vi "exercise7_readAI_samplesloop.vi"() -> ()   [LabVIEW 2018]
uses:
  <vilib>/DAQmx/read.llb/DAQmx Read (Analog Wfm 1Chan NSamp).vi
  <vilib>/DAQmx/create/channels.llb/DAQmx Create Channel (AI-Voltage-Basic).vi
  <vilib>/DAQmx/configure/timing.llb/DAQmx Timing (Sample Clock).vi
  <vilib>/DAQmx/miscellaneous.llb/DAQmx Fill In Error Info.vi
  <vilib>/express/express analysis/Spectral/Block/exnSpectralBlock spectral measurements RMS poly.vi
  <vilib>/express/express analysis/Spectral/Block/exnSpectralBlock spectral measurements RMS array WFM.vi
  <vilib>/express/express analysis/Spectral/XNode/ExpressSpectralMeasurementsBlockNode.xnode
panel:
  out "Waveform Chart (Pa)":waveform(dbl)(graph)
  out "FFT":cluster{"f0":dbl, "df":dbl, "magnitude":dbl[]}[](graph)
  in  "?":bool
  in  "maximum value":dbl=5.0
  in  "minimum value":dbl=-5.0
  in  "sample mode":i32(ring)=10123 items=["Finite Samples"=10178, "Continuous Samples"=10123, "Hardware Timed Single Point"=12522]
  in  "samples per channel":i32=40
  in  "rate":dbl=20.0
  out "error out":errorcluster
  out "Waveform Graph":waveform(dbl)(graph)
  out "Waveform Chart":waveform(dbl)(graph)
  in  "NI_channels":tag="Dev1/ai0"
  # "CANAL 0"
  # "CANAL 0"
  # "ACQUIRE SIGNAL (CONTINUOUS)"
  # "CHANNEL CONFIG"
  # "SAMPLING CONFIG"
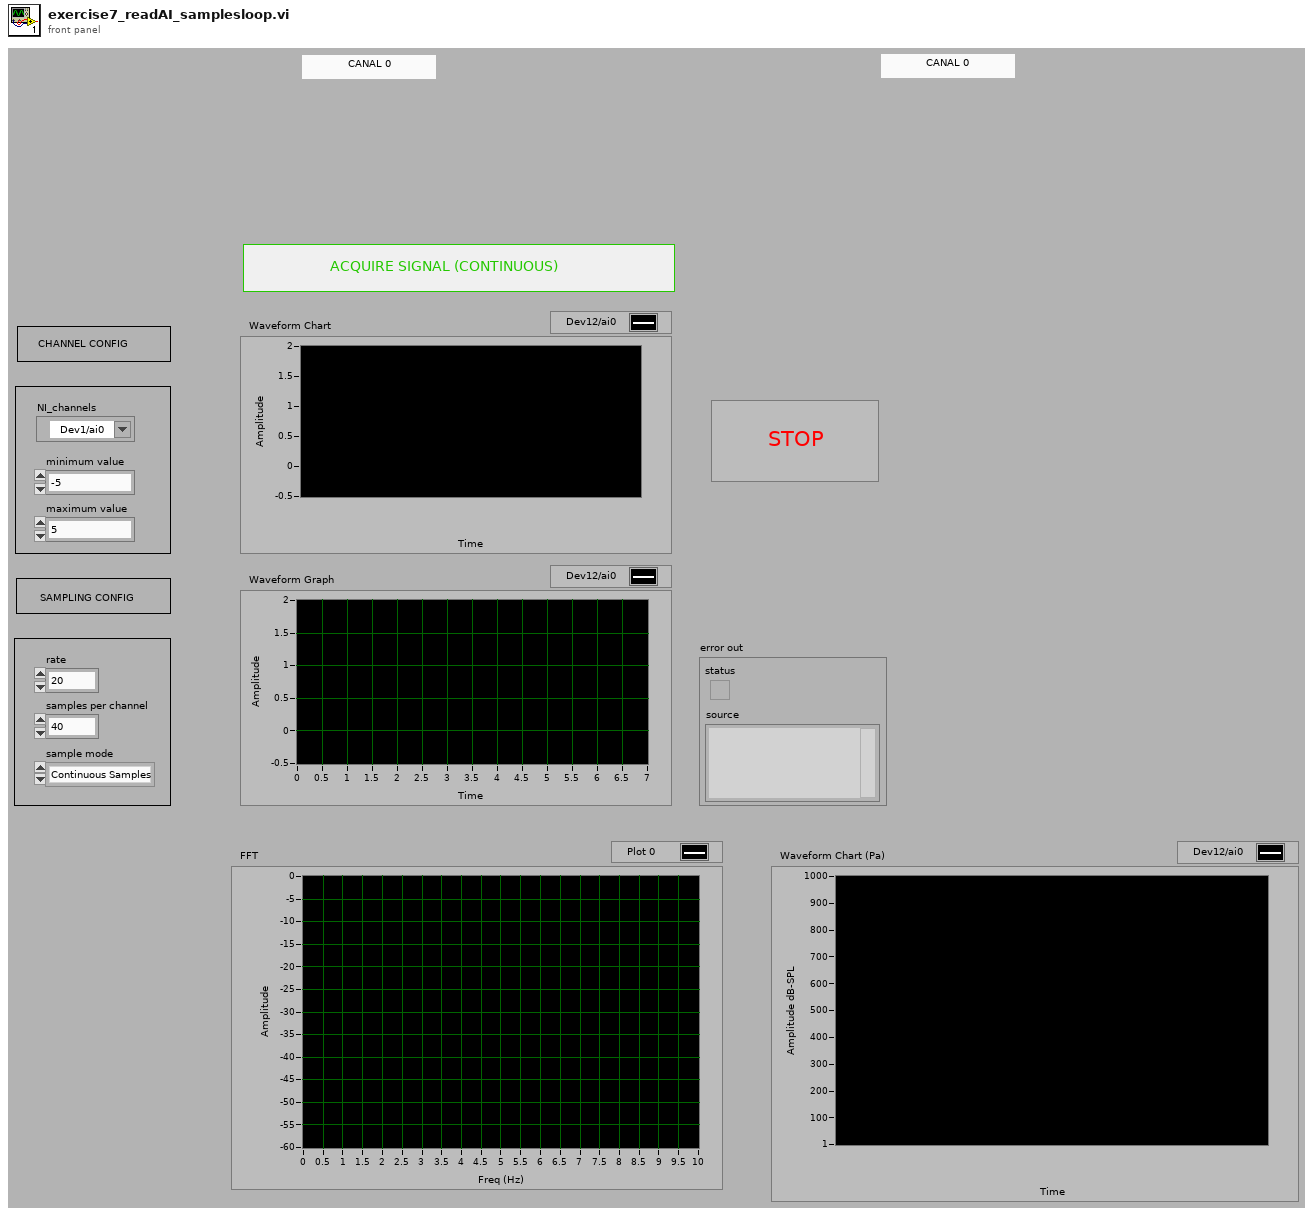
[diagram p1: front panel]
types:
  T1 = cluster{"averaging mode":u16, "weighting mode":u16, "number of averages":u32}
  T2 = cluster{"dB On (F)":bool, "unwrap phase (F)":bool, "convert to degree (F)":bool}
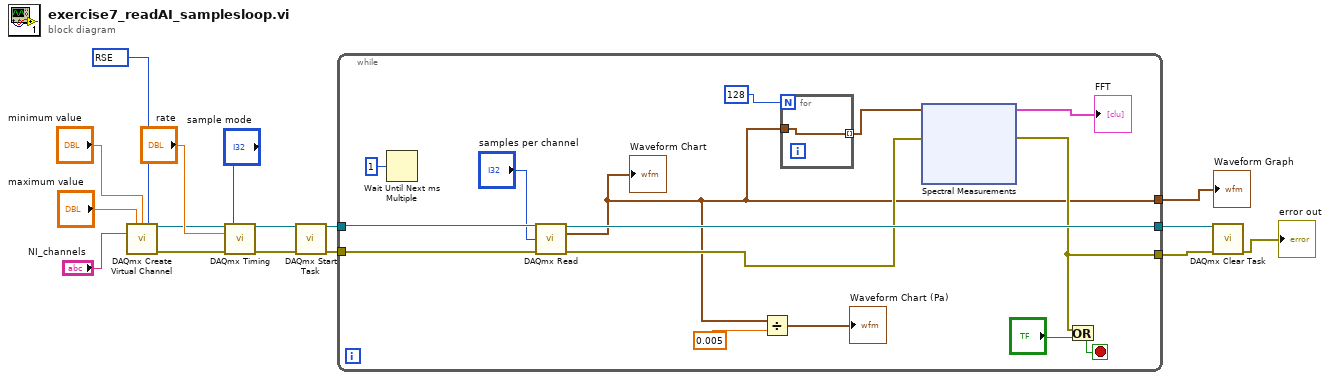
[diagram p0: block diagram]
diagram:
  w4 = 10083 items=["default"=-1, "RSE"=10083, "NRSE"=10078, "Differential"=10106, "Pseudodifferential"=12529] ("input terminal configuration")
  n1 = call-poly <vilib>:"DAQmx Create Virtual Channel.vi"("maximum value"="maximum value", "minimum value"="minimum value", "input terminal configuration"=w4, "physical channels"="NI_channels") -> ("task out"=w14:refnum<k21>, "error out"=w13:errorcluster)  [unwired: 10 in]
  n2 = call-poly <vilib>:"DAQmx Timing.vi"("task/channels in"=w14, "sample mode"="sample mode", "rate"="rate", "error in"=w13) -> ("task out"=w9:refnum<k21>, "error out"=w8:errorcluster)  [unwired: 10 in]
  n3 = call <vilib>:"DAQmx Start Task.vi"("task/channels in"=w9, "error in"=w8) -> ("task out"=w6:refnum<k21>, "error out"=w7:errorcluster)  [unwired: 12 in]
  n4 = while {
    tunnel: w7 -> [w31]
    tunnel: w6 -> [w30]
    tunnel: [w19] -> w3
    tunnel: [w29] -> w5
    tunnel: [w20] -> w2
    stop <- w26 stop-if-true
    n5 = Wait Until Next ms Multiple(millisecond multiple=u32 1) -> ()  [unwired: 1 out]
    n6 = call-poly <vilib>:"DAQmx Read.vi"("task/channels in"=w30, "number of samples per channel"="samples per channel", "error in"=w31) -> ("task out"=w29:refnum<k21>, "data"=w19:waveform(dbl), "error out"=w21:errorcluster)  [unwired: 10 in]
    "Waveform Chart" <- w19
    n7 = Divide(x=w19, y=0.005) -> (x/y=→"Waveform Chart (Pa)":waveform(dbl))
    n8 = for {
      N: 128 -> [_]
      tunnel: w19 -> [w32]
      tunnel: [w32] -> w23 mode=indexing
    }
    n9 = xnode "Spectral Measurements"("Signals"=w23, "error in (no error)"=w21) -> ("FFT - (RMS)"=→"FFT":cluster{"f0":dbl, "df":dbl, "magnitude":dbl[]}[], "error out"=w20:errorcluster)  [unwired: 1 out]
    n10 = Or(x=w20, y="?") -> (x .or. y?=w26:bool)
  }
  "Waveform Graph" <- w3
  n11 = call <vilib>:"DAQmx Clear Task.vi"("task in"=w5, "error in"=w2) -> ("error out"=→"error out":errorcluster)  [unwired: 13 in]
